vi "Write Version String.vi"(8 "error in (no error)":errorcluster, 10 "Version String":string, 11 "Splash Screen in":refnum<class "Splash Screen.lvclass">) -> (0 "error out":errorcluster, 3 "Splash Screen out":refnum<class "Splash Screen.lvclass">)   [LabVIEW 2015, in "Splash Screen.lvlib" / "Splash Screen.lvclass"]
uses:
  Splash Screen.lvclass
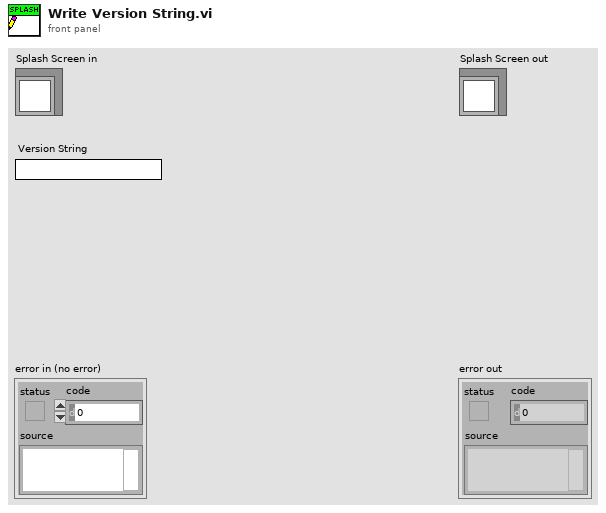
[diagram p1: front panel]
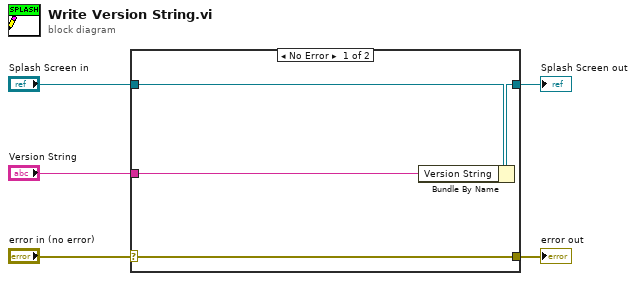
[diagram p0: block diagram]
diagram:
  n1 = case shown="No Error" "error in (no error)" {
    selector: "error in (no error)" -> [w9 w10]
    tunnel: [w9 w10] -> w4
    tunnel: [w7 w11] -> w2
    tunnel: "Splash Screen in" -> [w8 w11]
    tunnel: "Version String" -> [w6 _]
    frame No Error {
      n2 = Bundle By Name(cluster=w8, "Version String"=w6) -> (w7:refnum<class "Splash Screen.lvclass">)
    }
    frame Error {
    }
  }
  "error out" <- w4
  "Splash Screen out" <- w2
